vi "TODO Write time series JSON.vi"(0 "Client.lvclass in":refnum<class "Client.lvclass">, 5 "Database name":string, 7 "Precision":T1=enum."Nanoseconds", 11 "error in (no error)":errorcluster, 12 "JSON data":string) -> (4 "Client.lvclass out":refnum<class "Client.lvclass">, 15 "error out":errorcluster)   [LabVIEW 2018, in "InfluxDB Client.lvlib" / "Client.lvclass"]
doc: "Writes time series data (JSON format) to a specific database."
uses:
  Client.lvclass
  Controls/Precision.ctl
  Client.lvclass/Client.ctl
  <vilib>/httpClient/POSTBuffer.vi
  <vilib>/httpClient/LabVIEWHTTPClient.lvlib
  InfluxDB Client.lvlib
panel:
  out "Status":string
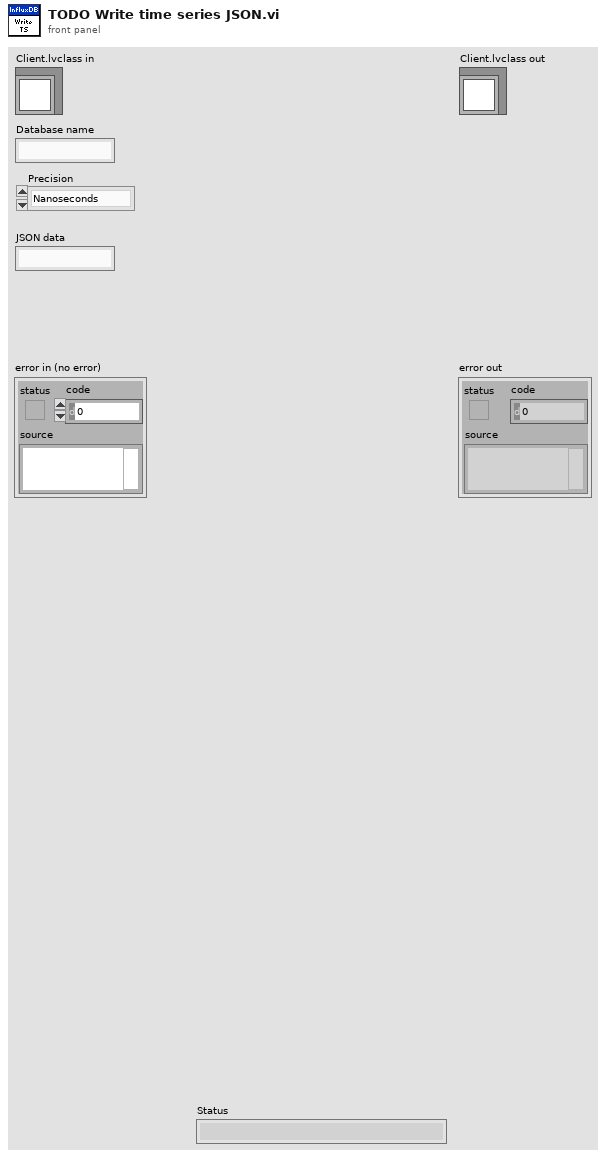
[diagram p1: front panel]
types:
  T1 = typedef "InfluxDB Client.lvlib/Precision.ctl" = enum16{"Seconds", "Milliseconds", "Nanoseconds"}
  T2 = typedef "LabVIEWHTTPClient.lvlib/ClientHandle.ctl" = refnum<k1>
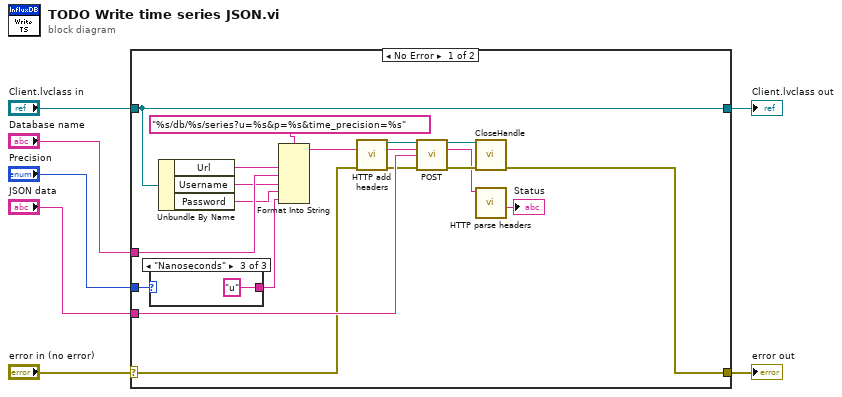
[diagram p0: block diagram]
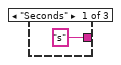
[diagram p2: hidden frame]
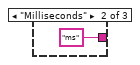
[diagram p3: hidden frame]
diagram:
  n1 = case shown="No Error" "error in (no error)" {
    selector: "error in (no error)" -> [w12 w30]
    tunnel: [w19 w30] -> w6
    tunnel: [w25 w29] -> w4
    tunnel: "Client.lvclass in" -> [w25 w29]
    tunnel: "Database name" -> [w16 _]
    tunnel: "Precision" -> [w9 _]
    tunnel: "JSON data" -> [w13 _]
    frame No Error {
      n2 = case shown="\"Nanoseconds\"" w9 {
        tunnel: ["s" ("Database name") "ms" ("Database name") "u" ("Database name")] -> w8
        frame "Seconds" {
        }
        frame "Milliseconds" {
        }
        frame "Nanoseconds" {
        }
      }
      n3 = Unbundle By Name(w25) -> ("Url"=w23:string, "Username"=w15:string, "Password"=w14:string)
      n4 = Format Into String(format string="%s/db/%s/series?u=%s&p=%s&time_precision=%s" ("url"), w23, w16, w15, w14, w8) -> (resulting string=w20:string)  [unwired: 2 in, 1 out]
      n5 = call "HTTP add headers.vi"("error in (no error)"=w12) -> ("client handle out"=w11:T2, "error out"=w10:errorcluster)  [unwired: 13 in]
      n6 = call-poly <vilib>:"POST.vi"("client handle"=w11, "url"=w20, "buffer"=w13, "error in (no error)"=w10) -> ("client handle out"=w22:T2, "headers"=w18:string, "error out"=w21:errorcluster)  [unwired: 8 in, 1 out]
      n7 = call <vilib>:"CloseHandle.vi"("client handle"=w22, "error in (no error)"=w21) -> ("error out"=w19:errorcluster)  [unwired: 13 in]
      n8 = call "HTTP parse headers.vi"("HTTP headers"=w18) -> ("Status"=→"Status":string)  [unwired: 7 in, 3 out]
    }
    frame Error {
    }
  }
  "error out" <- w6
  "Client.lvclass out" <- w4
